vi "oldAllyTeamToOOAllyTeam.vi"(5 "Side":enum16{"Esquerdo", "Direito"}(ring), 7 "Team":enum16{"Azul", "Amarelo"}(ring), 8 "error in (no error)":errorcluster, 10 "our_robots":T1[](array[typedef]), 11 "Ally in":refnum<class "Ally.lvclass">) -> (0 "error out":errorcluster, 3 "Ally out":refnum<class "Ally.lvclass">)   [LabVIEW 2023, in "Ally.lvclass"]
uses:
  Ally.lvclass
  Robot_class/Robot.lvclass
  Vision_class/Old vision/Controls/AI Robot.ctl
  Vision_class/Old vision/Controls/Functions Enum.ctl
  Vision_class/Old vision/Controls/AttackerStates.ctl
  Vision_class/Old vision/Controls/PathDests.ctl
  Vision_class/Old vision/Controls/PathDest.ctl
  Game_class/Navigation/VSSNavigation/VSSAttackerStates.ctl
  Team_class/Team.lvclass/Team.ctl
  Robot_class/roles.ctl
  Robot_class/Robot.lvclass/Robot.ctl
  Object_class/Object.lvclass/Object.ctl
  Robot_class/Write role.vi
  Object_class/Write x.vi
  Object_class/Write y.vi
  Robot_class/Write orientation.vi
  Robot_class/Write id.vi
  Robot_class/Write est_v_tang.vi
  Robot_class/Write est_v_norm.vi
  Object_class/Write pos_est_x.vi
  Object_class/Write pos_est_y.vi
  Team_class/Read RobotRef.vi
  Team_class/Write RobotRef.vi
panel:
  in  "Robot":refnum<class "Robot.lvclass">
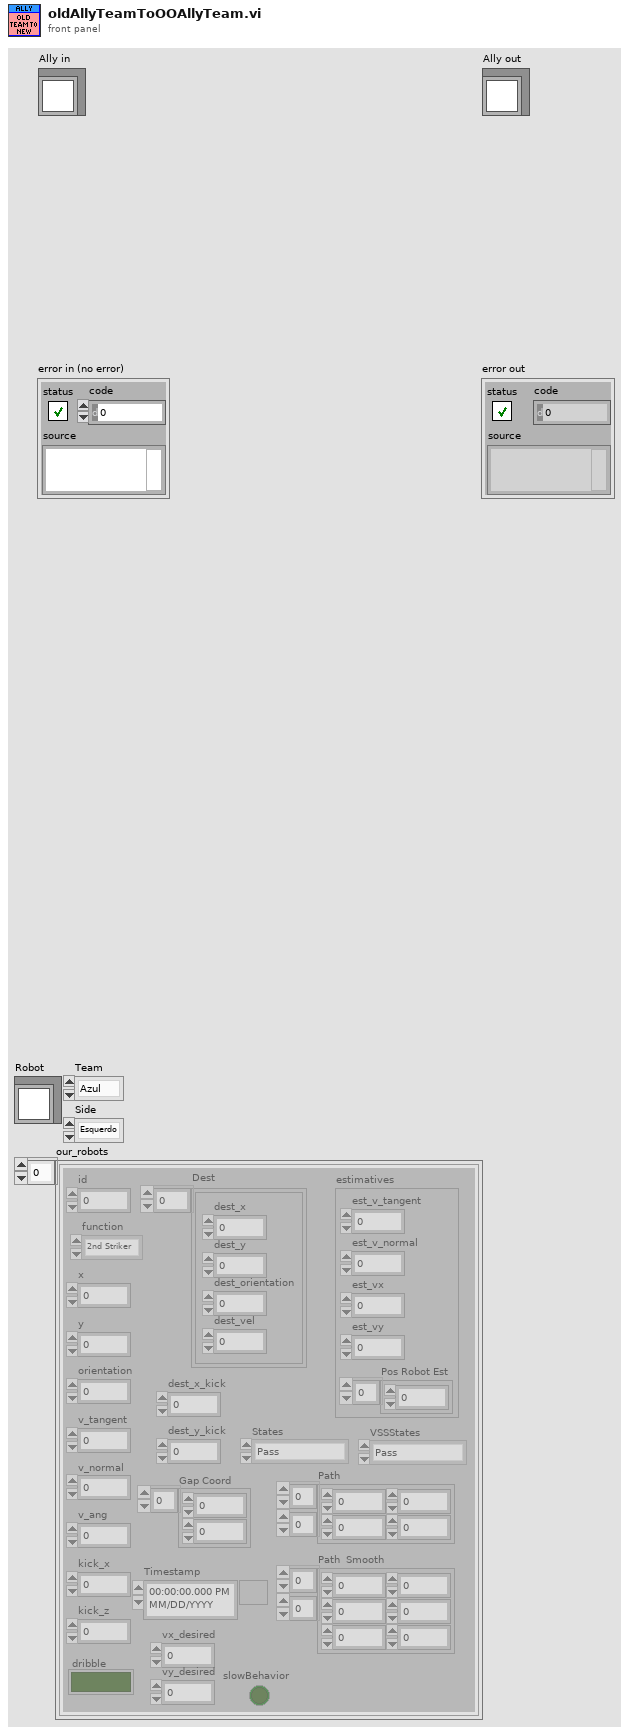
[diagram p1: front panel]
types:
  T1 = typedef "AI Robot.ctl" = cluster{"id":u32, "function":T2, "x":dbl, "y":dbl, "orientation":dbl, "v_tangent":dbl, "v_normal":dbl, "v_ang":dbl, "kick_x":dbl, "kick_z":dbl, "dribble":bool, "Timestamp":timestamp, "estimatives":cluster{"est_v_tangent":dbl, "est_v_normal":dbl, "est_vx":dbl, "est_vy":dbl, "Pos Robot Est":dbl[]}, "dest_x_kick":dbl, "dest_y_kick":dbl, "Gap Coord":dbl[], "States":T3, "Path ":dbl[][], "Path  Smooth":dbl[][], "Dest":T4, "vx_desired":dbl, "vy_desired":dbl, "slowBehavior":bool, "VSSStates":T6}
  T2 = typedef "Functions Enum.ctl" = enum16{"2nd Striker", "Attacker", "Goalie", "Defender", "Striker", "Goto 0", "Dummy", "Kicker", "ZigZag 0", "ZigZag 1", "ZigZag 2", "ZigZag 3", "ZigZag 4", "ZigZag 5", "ZigZag 6", "ZigZag 7", "ZigZag 8", ""}
  T3 = typedef "AttackerStates.ctl" = enum16{"Pass", "GoToTangent", "BallGetting", "GoToKick", ""}
  T4 = typedef "PathDests.ctl" = T5[]
  T5 = typedef "PathDest.ctl" = cluster{"dest_x":dbl, "dest_y":dbl, "dest_orientation":dbl, "dest_vel":dbl}
  T6 = typedef "VSSAttackerStates.ctl" = enum16{"Pass", "GoToTangent", "BallGetting", "GoToKick", "Rotate anti-clockwise", "Rotate Clockwise", ""}
  T7 = typedef "roles.ctl" = enum16{"BallChallengerAttackerVSS", "NormalAttackerVSS", "AttackerAimGoalVSS", "DefenderAreaVSS", "KeeperVSS", "Tabler", "TableFinalizer", "PrepareRollToPassRoller", "PrepareRollToPassReceiver", "SimplePassRoll", "SimplePassRollReceiver", "PenaltyDefense", "PreparePassReceiver 2", "PreparePassReceiver 1", "PassObserver", "Timeout", "Goto", "ZigZag", "None", "BallOutOfField", "DefenderArea", "Duelist", "AttackerStop", "FollowAttacker", "KeeperRole", "KickPenalty", "AttackerAimGoal", "AttackerBlock", "Marker", "Halt", "Shoot", "PassKicker", "PassReceiver", "TestRole", "PenaltyAttacker"}
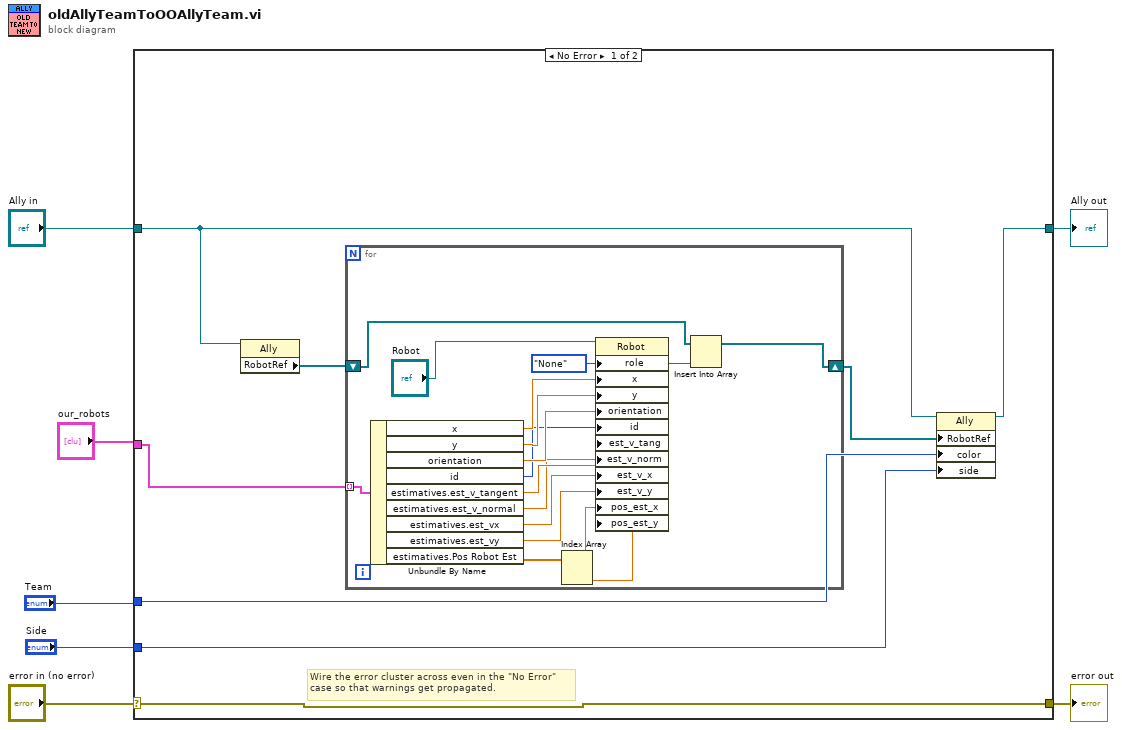
[diagram p0: block diagram]
diagram:
  n1 = case shown="No Error" "error in (no error)" {
    selector: "error in (no error)" -> [w15 w34]
    tunnel: [w15 w34] -> w6
    tunnel: [w12 w33] -> w4
    tunnel: "Ally in" -> [w9 w33]
    tunnel: "our_robots" -> [w14 _]
    tunnel: "Team" -> [w11 _]
    tunnel: "Side" -> [w10 _]
    frame No Error {
      # "Wire the error cluster across even in the \"No Error\"\ncase so that warnings get propagated."
      n2 = property class="Ally"(reference=w9) -> ("RobotRef"=w13:refnum<class "Robot.lvclass">[])  [unwired: 1 in, 2 out]
      n3 = for {
        tunnel: w14 -> [w32] mode=indexing
        shift-right: [w24] -> w8
        shift-left: w13 -> [w26]
        n4 = Unbundle By Name(w32) -> ("x"=w30:dbl, "y"=w29:dbl, "orientation"=w28:dbl, "id"=w27:u32, "estimatives.est_v_tangent"=w23:dbl, "estimatives.est_v_normal"=w22:dbl, "estimatives.est_vx"=w21:dbl, "estimatives.est_vy"=w20:dbl, "estimatives.Pos Robot Est"=w19:dbl[])
        n5 = Index Array(array=w19) -> (element #1=w18:dbl, element #2=w17:dbl)  [unwired: 2 in]
        n6 = property class="Robot"(reference="Robot", "role"=roles."None", "x"=w30, "y"=w29, "orientation"=w28, "id"=w27, "est_v_tang"=w23, "est_v_norm"=w22, "est_v_x"=w21, "est_v_y"=w20, "pos_est_x"=w18, "pos_est_y"=w17) -> (reference out=w25:refnum<class "Robot.lvclass">)  [unwired: 1 in, 1 out]
        n7 = Insert Into Array(array=w26, new element=w25) -> (w24:refnum<class "Robot.lvclass">[])  [unwired: 1 in]
      }
      n8 = property class="Ally"(reference=w9, "RobotRef"=w8, "color"=w11, "side"=w10) -> (reference out=w12:refnum<class "Ally.lvclass">)  [unwired: 1 in, 1 out]
    }
    frame Error {
    }
  }
  "error out" <- w6
  "Ally out" <- w4
